vi "Presentation LabVIEW.vi"() -> ()   [LabVIEW 2020]
panel:
  out "Led Boucle":bool
  out "Itérateur":i32
  out "longueur":i32
  out "Indicateur Chaîne":string
  out "Indicateur Booléen":bool
  out "Indicateur Numérique":dbl
  in  "Commande Chaîne":string
  in  "Commande Bouton":bool
  in  "Commande Numérique":dbl
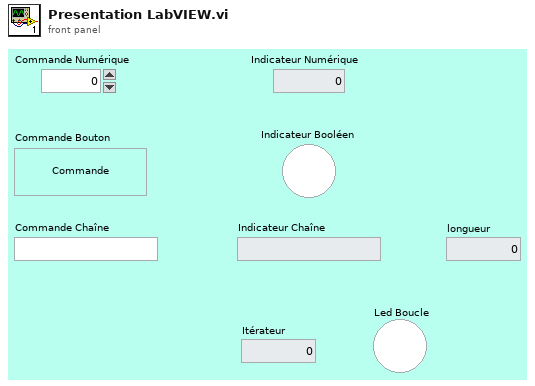
[diagram p1: front panel]
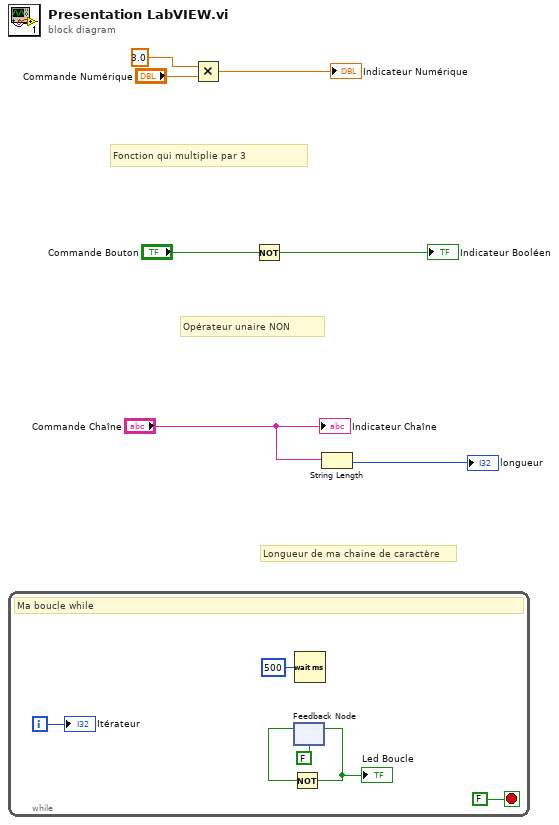
[diagram p0: block diagram]
diagram:
  # "Longueur de ma chaine de caractère"
  # "Opérateur unaire NON"
  # "Fonction qui multiplie par 3"
  n1 = while {
    i -> [w12]
    stop <- FALSE stop-if-true
    # "Ma boucle while"
    n2 = feedback #1(FALSE) -> (w9:bool)
    n3 = Not(x=w9) -> (.not. x?=w10:bool)
    "Led Boucle" <- w10
    n4 = feedback-in #1(w10) -> ()
    n5 = Wait (ms)(milliseconds to wait=u32 500 ("attente (ms)")) -> ()  [unwired: 1 out]
    "Itérateur" <- w12
  }
  n6 = Multiply(x=3.0, y="Commande Numérique") -> (x*y=→"Indicateur Numérique":dbl)
  n7 = Not(x="Commande Bouton") -> (.not. x?=→"Indicateur Booléen":bool)
  n8 = String Length(string="Commande Chaîne") -> (length=→"longueur":i32)
  "Indicateur Chaîne" <- "Commande Chaîne"
